vi "GraphForm (SubVI) 16.vi"() -> ()   [LabVIEW 2013]
uses:
  Global R.vi
  Global T.vi
panel:
  in  "9_ch_visible":bool=TRUE
  out "T15":dbl format="%.2f"
  out "T13":dbl format="%.2f"
  out "T16":dbl format="%.2f"
  out "T14":dbl format="%.2f"
  out "T11":dbl format="%.2f"
  out "T9":dbl format="%.2f"
  out "T12":dbl format="%.2f"
  out "T10":dbl format="%.2f"
  in  "10_ch_visible":bool=TRUE
  in  "11_ch_visible":bool=TRUE
  in  "12_ch_visible":bool=TRUE
  in  "13_ch_visible":bool=TRUE
  in  "14_ch_visible":bool=TRUE
  in  "15_ch_visible":bool=TRUE
  in  "16_ch_visible":bool=TRUE
  in  "1_ch_visible":bool=TRUE
  out "T7":dbl format="%.2f"
  out "T5":dbl format="%.2f"
  out "T8":dbl format="%.2f"
  out "T6":dbl format="%.2f"
  out "T3":dbl format="%.2f"
  out "T1":dbl format="%.2f"
  out "T4":dbl format="%.2f"
  out "T2":dbl format="%.2f"
  in  "R":T1
  in  "stop":bool
  in  "T":T2
  in  "Title":string
  out "часы":string="0"
  in  "Добавить время":dbl(ring)=300.0 items=["1 мин."=60.0, "5 мин."=300.0, "20 мин."=1200.0]
  out "мин.":string="1"
  in  "xScale +":bool
  in  "xScale -":bool
  in  "Autoscale":bool=TRUE
  in  "R max":u16=6000 min=2 max=10000 step=1
  in  "R min":u16=100 min=1 max=350
  in  "Т max":u16=300 min=2 max=500 step=1
  in  "Т min":u16=3 min=1 max=350
  in  "2_ch_visible":bool=TRUE
  in  "3_ch_visible":bool=TRUE
  in  "4_ch_visible":bool=TRUE
  in  "5_ch_visible":bool=TRUE
  in  "6_ch_visible":bool=TRUE
  in  "7_ch_visible":bool=TRUE
  in  "8_ch_visible":bool=TRUE
  out "Graphs T":dynamicdata(graph)
  out "Graphs R":dynamicdata(graph)
  # "№"
  # "№"
  # "T [К]"
  # "T [К]"
  # "1"
  # "9"
  # "2"
  # "10"
  # "3"
  # "11"
  # "4"
  # "12"
  # "5"
  # "13"
  # "6"
  # "14"
  # "7"
  # "15"
  # "8"
  # "16"
  # "Интервал просмотра"
  # ":"
  # "Шкала R"
  # "Шкала Т"
  # "Температура, К"
  # "Сопротивление, Ом"
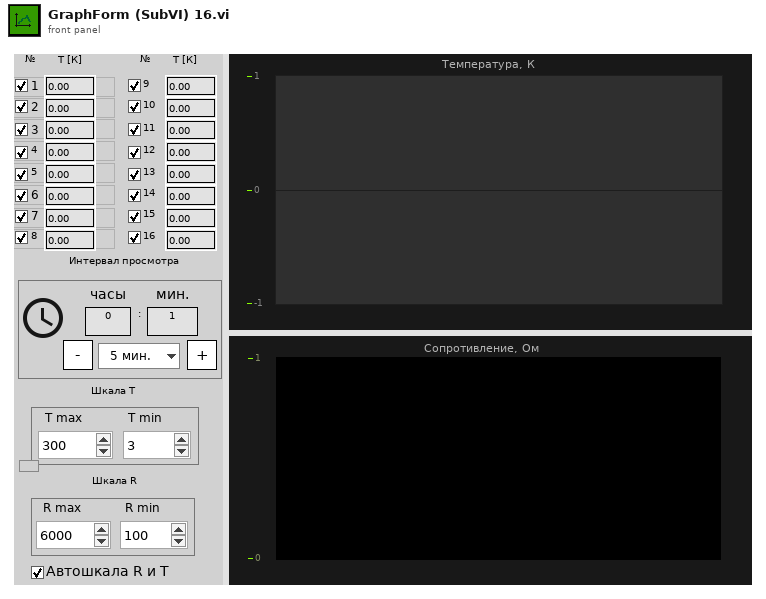
[diagram p1: front panel]
types:
  T1 = cluster{" R1":dbl, " R2":dbl, " R3":dbl, " R4":dbl, " R5":dbl, "R6":dbl, " R7":dbl, "R8":dbl, "R16":dbl, " R15":dbl, "R14":dbl, " R13":dbl, " R12":dbl, " R11":dbl, " R10":dbl, " R9":dbl}
  T2 = cluster{" T1":dbl, " T2":dbl, " T3":dbl, " T4":dbl, " T5":dbl, "T6":dbl, " T7":dbl, "T8":dbl, "T16":dbl, " T15":dbl, "T14":dbl, " T13":dbl, " T12":dbl, " T11":dbl, " T10":dbl, " T9":dbl}
  T3 = cluster{"1":dbl, " 2":dbl, " 3":dbl, "4":dbl, "5":dbl, "6":dbl, "7":dbl, "8":dbl, "9":dbl, " 10":dbl, " 11":dbl, "12":dbl, "13":dbl, "14":dbl, "15":dbl, "16":dbl}
  T4 = cluster{bool, bool, bool, bool, bool, bool, bool, bool, bool, bool, bool, bool, bool, bool, bool, bool}
  T5 = typedef "LVDateTimeRec.ctl" = cluster{"fractional second":dbl, "second":i32, "minute":i32, "hour":i32, "day of month":i32, "month":i32, "year":i32, "day of week":i32, "day of year":i32, "DST":i32}
  T6 = cluster{"1":dbl, " 2":dbl, " 3":dbl, "4":dbl, "5":dbl, "6":dbl, "7":dbl, "8":dbl, "1 2":dbl, " 10":dbl, " 11":dbl, "12":dbl, "13":dbl, "14":dbl, "15":dbl, "16":dbl}
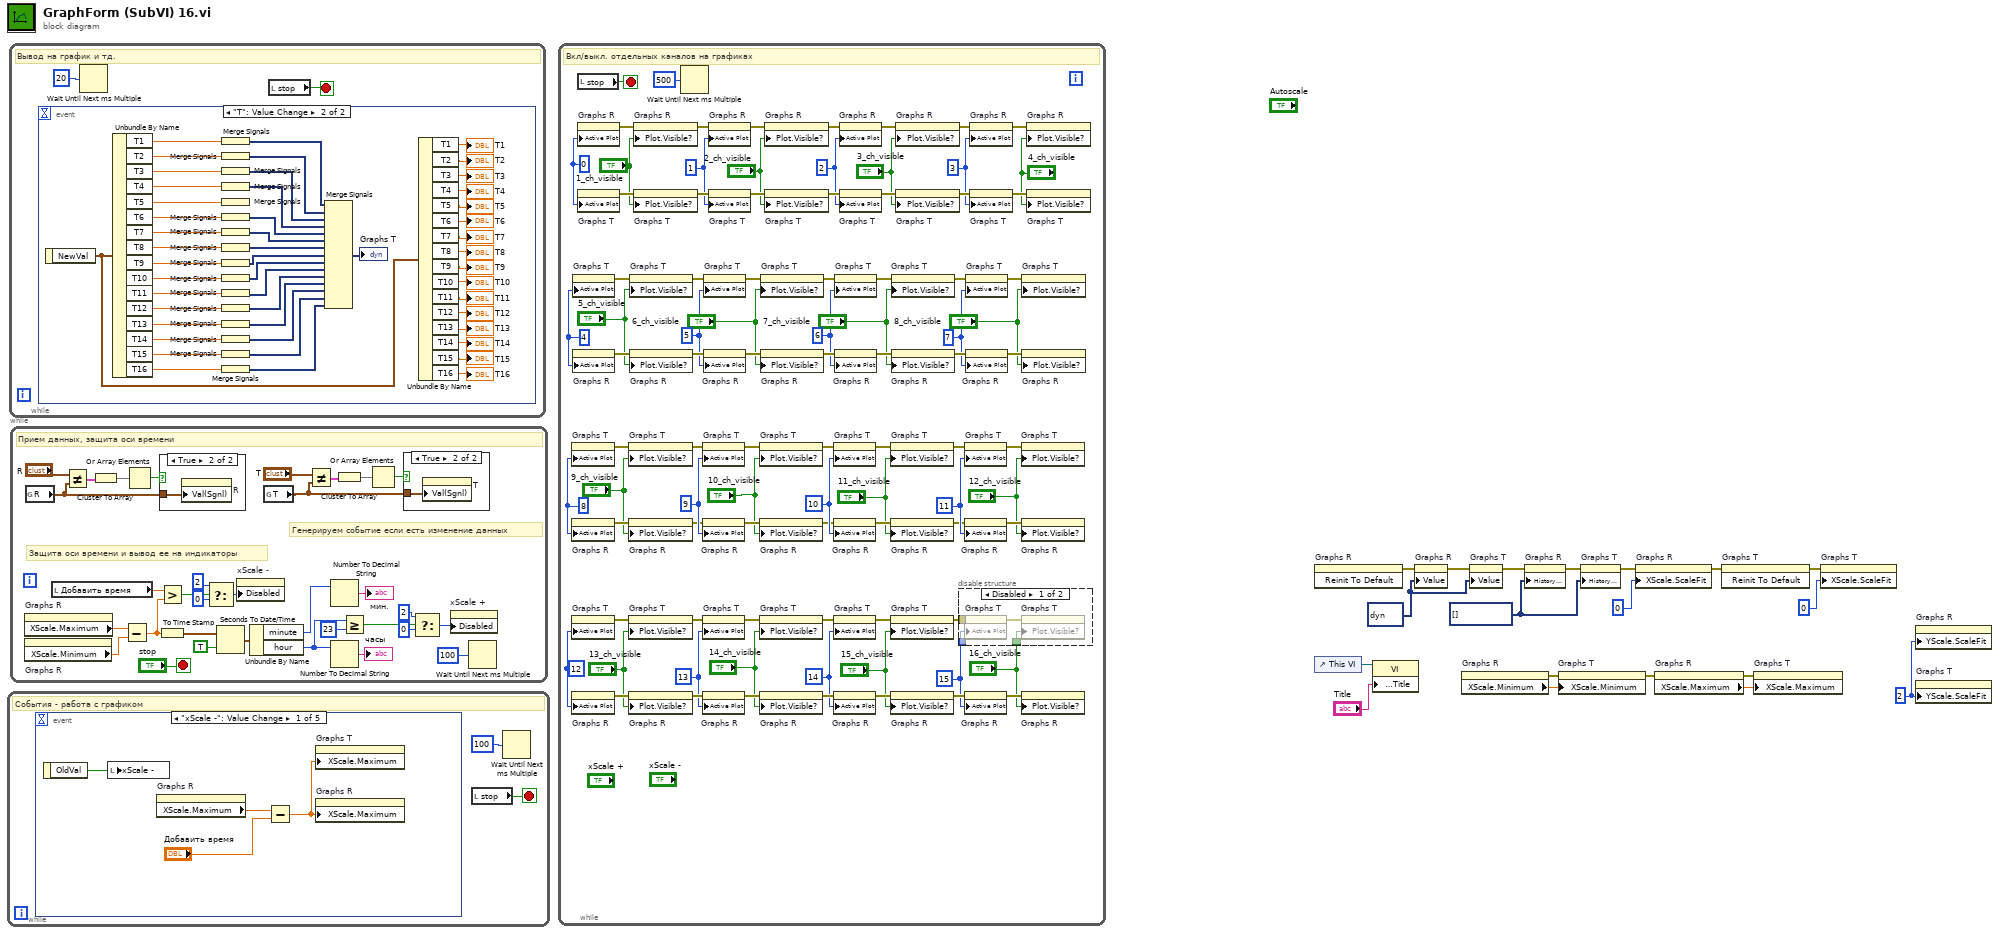
[diagram p0: block diagram]
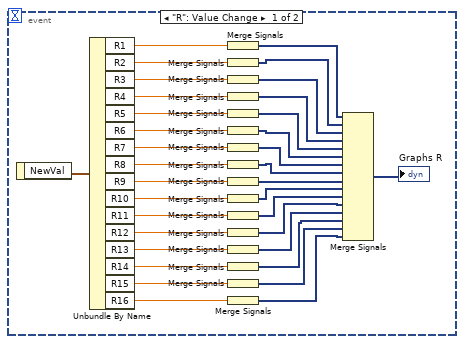
[diagram p3: hidden frame]
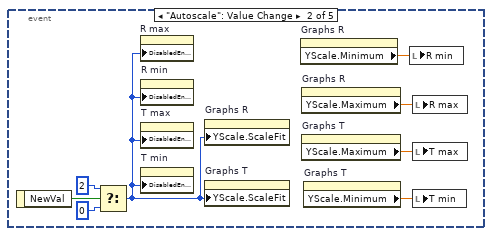
[diagram p6: hidden frame]
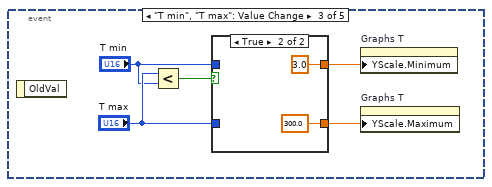
[diagram p7: hidden frame]
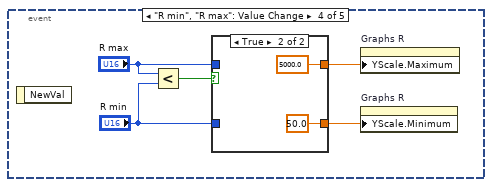
[diagram p9: hidden frame]
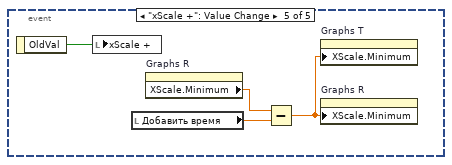
[diagram p11: hidden frame]
diagram:
  w3 = u8 2 ("Y Scale.Scale Fit")
  w14 = dynamicdata[] [] ("History Data")
  w15 = dynamicdata [{"t0"=timestamp(3465273261.7246556 s since 1904-01-01), "dt"=1.0, "Y"=[0.1931097262457384]}, {"t0"=timestamp(3465273261.7246556 s since 1904-01-01), "dt"=1.0, "Y"=[0.3594116459482981]}, {"t0"=timestamp(3465273261.7246556 s since 1904-01-01), "dt"=1.0, "Y"=[0.8898205452798131]}, {"t0"=timestamp(3465273261.7246556 s since 1904-01-01), "dt"=1.0, "Y"=[0.747699236883661]}] ("Graphs")
  n1 = while {
    stop <- w20 stop-if-true
    # "События - работа с графиком"
    n2 = event shown="[0] \"xScale -\": Value Change" {
      selector: _ -> [_ _ _ _ _]
      dyn-events: _ -> [_ _ _ _ _]
      timeout: _ -> [_ _ _ _ _]
      event "xScale -": Value Change {
        n3 = event-data() -> ("OldVal"=w25:bool)  [unwired: 1 in]
        n4 = local write "xScale -"(w25) -> ()
        n5 = property on="Graphs R" class="WFChart (strict)"() -> ("XScale.Maximum"=w23:dbl)  [unwired: 2 in, 2 out]
        n6 = Subtract(x=w23, y="Добавить время") -> (x-y=w24:dbl)
        n7 = property on="Graphs T" class="WFChart (strict)"("XScale.Maximum"=w24) -> ()  [unwired: 2 in, 2 out]
        n8 = property on="Graphs R" class="WFChart (strict)"("XScale.Maximum"=w24) -> ()  [unwired: 2 in, 2 out]
      }
      event "Autoscale": Value Change {
        n9 = event-data() -> ("NewVal"=w26:bool)  [unwired: 1 in]
        n10 = Select(t=u8 2 ("Y Scale.Scale Fit"), s=w26, f=u8 0 ("Y Scale.Scale Fit")) -> (s? t:f=w29:u8)
        n11 = property on="R max" class="DigNum (strict)"("DisabledEnum"=w29) -> ()  [unwired: 2 in, 2 out]
        n12 = property on="R min" class="DigNum (strict)"("DisabledEnum"=w29) -> ()  [unwired: 2 in, 2 out]
        n13 = property on="Т max" class="DigNum (strict)"("DisabledEnum"=w29) -> ()  [unwired: 2 in, 2 out]
        n14 = property on="Т min" class="DigNum (strict)"("DisabledEnum"=w29) -> ()  [unwired: 2 in, 2 out]
        n15 = property on="Graphs R" class="WFChart (strict)"("YScale.ScaleFit"=w29) -> ()  [unwired: 2 in, 2 out]
        n16 = property on="Graphs T" class="WFChart (strict)"("YScale.ScaleFit"=w29) -> ()  [unwired: 2 in, 2 out]
        n17 = property on="Graphs R" class="WFChart (strict)"() -> ("YScale.Minimum"=w30:dbl)  [unwired: 2 in, 2 out]
        n18 = property on="Graphs R" class="WFChart (strict)"() -> ("YScale.Maximum"=w31:dbl)  [unwired: 2 in, 2 out]
        n19 = property on="Graphs T" class="WFChart (strict)"() -> ("YScale.Maximum"=w33:dbl)  [unwired: 2 in, 2 out]
        n20 = property on="Graphs T" class="WFChart (strict)"() -> ("YScale.Minimum"=w32:dbl)  [unwired: 2 in, 2 out]
        n21 = local write "R min"(w30) -> ()
        n22 = local write "R max"(w31) -> ()
        n23 = local write "Т max"(w33) -> ()
        n24 = local write "Т min"(w32) -> ()
      }
      event "Т min", "Т max": Value Change {
        n25 = event-data() -> ()  [unwired: 1 in, 1 out]
        n26 = Less?(x="Т max", y="Т min") -> (x < y?=w36:bool)
        n27 = case shown="True" w36 {
          tunnel: [w39 300.0 ("x+1")] -> w38
          tunnel: [w40 3.0 ("x+1")] -> w37
          tunnel: "Т max" -> [w39 _]
          tunnel: "Т min" -> [w40 _]
          frame False {
          }
          frame True {
          }
        }
        n28 = property on="Graphs T" class="WFChart (strict)"("YScale.Minimum"=w37) -> ()  [unwired: 2 in, 2 out]
        n29 = property on="Graphs T" class="WFChart (strict)"("YScale.Maximum"=w38) -> ()  [unwired: 2 in, 2 out]
      }
      event "R min", "R max": Value Change {
        n30 = event-data() -> ()  [unwired: 1 in, 1 out]
        n31 = Less?(x="R max", y="R min") -> (x < y?=w47:bool)
        n32 = case shown="True" w47 {
          tunnel: [w48 5000.0 ("x+1")] -> w43
          tunnel: [w49 50.0 ("x+1")] -> w44
          tunnel: "R max" -> [w48 _]
          tunnel: "R min" -> [w49 _]
          frame False {
          }
          frame True {
          }
        }
        n33 = property on="Graphs R" class="WFChart (strict)"("YScale.Maximum"=w43) -> ()  [unwired: 2 in, 2 out]
        n34 = property on="Graphs R" class="WFChart (strict)"("YScale.Minimum"=w44) -> ()  [unwired: 2 in, 2 out]
      }
      event "xScale +": Value Change {
        n35 = event-data() -> ("OldVal"=w55:bool)  [unwired: 1 in]
        n36 = local write "xScale +"(w55) -> ()
        n37 = local read "Добавить время"() -> (w52:dbl)
        n38 = property on="Graphs R" class="WFChart (strict)"() -> ("XScale.Minimum"=w53:dbl)  [unwired: 2 in, 2 out]
        n39 = Subtract(x=w53, y=w52) -> (x-y=w54:dbl)
        n40 = property on="Graphs T" class="WFChart (strict)"("XScale.Minimum"=w54) -> ()  [unwired: 2 in, 2 out]
        n41 = property on="Graphs R" class="WFChart (strict)"("XScale.Minimum"=w54) -> ()  [unwired: 2 in, 2 out]
      }
    }
    n42 = local read "stop"() -> (w20:bool)
    n43 = Wait Until Next ms Multiple(millisecond multiple=u32 100) -> ()  [unwired: 1 out]
  }
  n44 = while {
    stop <- w56 stop-if-true
    # "Вывод на график и тд."
    n45 = event shown="[1] \"T\": Value Change" {
      selector: _ -> [_ _]
      dyn-events: _ -> [_ _]
      timeout: _ -> [_ _]
      event "R": Value Change {
        n46 = event-data() -> ("NewVal"=w91:T1)  [unwired: 1 in]
        n47 = Unbundle By Name(w91) -> ("R1"=w90:dbl, "R2"=w89:dbl, "R3"=w88:dbl, "R4"=w87:dbl, "R5"=w86:dbl, "R6"=w85:dbl, "R7"=w84:dbl, "R8"=w83:dbl, "R9"=w82:dbl, "R10"=w81:dbl, "R11"=w80:dbl, "R12"=w79:dbl, "R13"=w78:dbl, "R14"=w77:dbl, "R15"=w76:dbl, "R16"=w75:dbl)
        n48 = Merge Signals(w90) -> (w74:dynamicdata)
        n49 = Merge Signals(w89) -> (w73:dynamicdata)
        n50 = Merge Signals(w88) -> (w72:dynamicdata)
        n51 = Merge Signals(w87) -> (w71:dynamicdata)
        n52 = Merge Signals(w86) -> (w70:dynamicdata)
        n53 = Merge Signals(w85) -> (w69:dynamicdata)
        n54 = Merge Signals(w84) -> (w68:dynamicdata)
        n55 = Merge Signals(w83) -> (w67:dynamicdata)
        n56 = Merge Signals(w82) -> (w66:dynamicdata)
        n57 = Merge Signals(w81) -> (w65:dynamicdata)
        n58 = Merge Signals(w80) -> (w64:dynamicdata)
        n59 = Merge Signals(w79) -> (w63:dynamicdata)
        n60 = Merge Signals(w78) -> (w62:dynamicdata)
        n61 = Merge Signals(w77) -> (w61:dynamicdata)
        n62 = Merge Signals(w76) -> (w60:dynamicdata)
        n63 = Merge Signals(w75) -> (w59:dynamicdata)
        n64 = Merge Signals(w74, w73, w72, w71, w70, w69, w68, w67, w66, w65, w64, w63, w62, w61, w60, w59) -> (→"Graphs R":dynamicdata)
      }
      event "T": Value Change {
        n65 = event-data() -> ("NewVal"=w108:T2)  [unwired: 1 in]
        n66 = Unbundle By Name(w108) -> ("T1"=w140:dbl, "T2"=w139:dbl, "T3"=w138:dbl, "T4"=w137:dbl, "T5"=w136:dbl, "T6"=w135:dbl, "T7"=w134:dbl, "T8"=w133:dbl, "T9"=w132:dbl, "T10"=w131:dbl, "T11"=w130:dbl, "T12"=w129:dbl, "T13"=w128:dbl, "T14"=w127:dbl, "T15"=w126:dbl, "T16"=w125:dbl)
        n67 = Merge Signals(w140) -> (w124:dynamicdata)
        n68 = Merge Signals(w139) -> (w123:dynamicdata)
        n69 = Merge Signals(w138) -> (w112:dynamicdata)
        n70 = Merge Signals(w137) -> (w122:dynamicdata)
        n71 = Merge Signals(w136) -> ()  [unwired: 1 out]
        n72 = Merge Signals(w135) -> (w121:dynamicdata)
        n73 = Merge Signals(w134) -> (w120:dynamicdata)
        n74 = Merge Signals(w133) -> (w119:dynamicdata)
        n75 = Merge Signals(w132) -> (w118:dynamicdata)
        n76 = Merge Signals(w131) -> (w117:dynamicdata)
        n77 = Merge Signals(w130) -> (w111:dynamicdata)
        n78 = Merge Signals(w129) -> (w110:dynamicdata)
        n79 = Merge Signals(w128) -> (w116:dynamicdata)
        n80 = Merge Signals(w127) -> (w115:dynamicdata)
        n81 = Merge Signals(w126) -> (w114:dynamicdata)
        n82 = Merge Signals(w125) -> (w113:dynamicdata)
        n83 = Merge Signals(w124, w123, w112, w122, w121, w120, w119, w118, w117, w111, w110, w116, w115, w114, w113) -> (→"Graphs T":dynamicdata)
        n84 = Unbundle By Name(w108) -> ("T1"=→"T1":dbl, "T2"=→"T2":dbl, "T3"=→"T3":dbl, "T4"=→"T4":dbl, "T5"=→"T5":dbl, "T6"=→"T6":dbl, "T7"=→"T7":dbl, "T8"=→"T8":dbl, "T9"=→"T9":dbl, "T10"=→"T10":dbl, "T11"=→"T11":dbl, "T12"=→"T12":dbl, "T13"=→"T13":dbl, "T14"=→"T14":dbl, "T15"=→"T15":dbl, "T16"=→"T16":dbl)
      }
    }
    n85 = Wait Until Next ms Multiple(millisecond multiple=u32 20) -> ()  [unwired: 1 out]
    n86 = local read "stop"() -> (w56:bool)
  }
  n87 = while {
    stop <- "stop" stop-if-true
    # "Генерируем событие если есть изменение данных"
    # "Защита оси времени и вывод ее на индикаторы"
    # "Прием данных, защита оси времени"
    n88 = property on="Graphs R" class="WFChart (strict)"() -> ("XScale.Maximum"=w172:dbl)  [unwired: 2 in, 2 out]
    n89 = property on="Graphs R" class="WFChart (strict)"() -> ("XScale.Minimum"=w171:dbl)  [unwired: 2 in, 2 out]
    n90 = global read "Global R.vi" "R"() -> (w158:T3)
    n91 = local read "Добавить время"() -> (w170:dbl)
    n92 = Not Equal?(x="R", y=w158) -> (x != y?=w155:T4)
    n93 = Cluster To Array(cluster=w155) -> (array=w156:bool[])
    n94 = Subtract(x=w172, y=w171) -> (x-y=w165:dbl)
    n95 = Or Array Elements(Boolean array=w156) -> (logical OR=w157:bool)
    n96 = Greater?(x=w170, y=w165) -> (0:w154:bool)
    n97 = To Time Stamp(1:w165) -> (0:w168:timestamp)
    n98 = case shown="True" w157 {
      tunnel: w158 -> [_ w174]
      frame False {
      }
      frame True {
        n99 = property on="R" class="Clust (strict)"("Val(Sgnl)"=w174) -> ()  [unwired: 2 in, 2 out]
      }
    }
    n100 = Select(t=u8 2 ("Disabled"), s=w154, f=u8 0 ("Disabled")) -> (s? t:f=w153:u8)
    n101 = Seconds To Date/Time(time stamp (now)=w168, to UTC (F)=TRUE) -> (date time rec=w167:T5)
    n102 = property on="xScale -" class="Bool (strict)"("Disabled"=w153) -> ()  [unwired: 2 in, 2 out]
    n103 = Unbundle By Name(w167) -> ("minute"=w166:i32, "hour"=w164:i32)
    n104 = global read "Global T.vi" "T"() -> (w141:T6)
    n105 = Not Equal?(x="T", y=w141) -> (x != y?=w146:T4)
    n106 = Number To Decimal String(number=w166) -> (decimal integer string=→"мин.":string)  [unwired: 1 out]
    n107 = Number To Decimal String(number=w164) -> (decimal integer string=→"часы":string)  [unwired: 1 out]
    n108 = Cluster To Array(cluster=w146) -> (array=w145:bool[])
    n109 = Greater Or Equal?(x=w164, y=23) -> (x >= y?=w149:bool)
    n110 = Or Array Elements(Boolean array=w145) -> (logical OR=w144:bool)
    n111 = case shown="True" w144 {
      tunnel: w141 -> [_ w173]
      frame False {
      }
      frame True {
        n112 = property on="T" class="Clust (strict)"("Val(Sgnl)"=w173) -> ()  [unwired: 2 in, 2 out]
      }
    }
    n113 = Select(t=u8 2 ("Disabled"), s=w149, f=u8 0 ("Disabled")) -> (s? t:f=w147:u8)
    n114 = property on="xScale +" class="Bool (strict)"("Disabled"=w147) -> ()  [unwired: 2 in, 2 out]
    n115 = Wait Until Next ms Multiple(millisecond multiple=u32 100) -> ()  [unwired: 1 out]
  }
  n116 = while {
    stop <- w218 stop-if-true
    w180 = u32 15 ("Active Plot")
    w181 = u32 14 ("Active Plot")
    w182 = u32 13 ("Active Plot")
    w179 = u32 12 ("Active Plot")
    w217 = u32 11 ("Active Plot")
    w216 = u32 10 ("Active Plot")
    w215 = u32 9 ("Active Plot")
    w214 = u32 8 ("Active Plot")
    w220 = u32 7 ("Active Plot")
    w222 = u32 6 ("Active Plot")
    w224 = u32 5 ("Active Plot")
    w226 = u32 4 ("Active Plot")
    w236 = u32 3 ("Active Plot")
    w239 = u32 2 ("Active Plot")
    w242 = u32 1 ("Active Plot")
    w247 = u32 0 ("Active Plot")
    # "Вкл/выкл. отдельных каналов на графиках"
    n117 = property on="Graphs T" class="WFChart (strict)"("Active Plot"=w214) -> (error out=w200:errorcluster)  [unwired: 2 in, 1 out]
    n118 = property on="Graphs R" class="WFChart (strict)"("Active Plot"=w214) -> (error out=w213:errorcluster)  [unwired: 2 in, 1 out]
    n119 = property on="Graphs T" class="WFChart (strict)"("Active Plot"=w179) -> (error out=w195:errorcluster)  [unwired: 2 in, 1 out]
    n120 = property on="Graphs R" class="WFChart (strict)"("Active Plot"=w179) -> (error out=w183:errorcluster)  [unwired: 2 in, 1 out]
    n121 = property on="Graphs T" class="WFChart (strict)"("Active Plot"=w226) -> (error out=w258:errorcluster)  [unwired: 2 in, 1 out]
    n122 = property on="Graphs R" class="WFChart (strict)"("Active Plot"=w226) -> (error out=w227:errorcluster)  [unwired: 2 in, 1 out]
    n123 = local read "stop"() -> (w218:bool)
    n124 = property on="Graphs R" class="WFChart (strict)"("Active Plot"=w247) -> (error out=w248:errorcluster)  [unwired: 2 in, 1 out]
    n125 = property on="Graphs T" class="WFChart (strict)"("Active Plot"=w247) -> (error out=w259:errorcluster)  [unwired: 2 in, 1 out]
    n126 = property on="Graphs T" class="WFChart (strict)"(error in=w200, "Plot.Visible?"="9_ch_visible") -> (error out=w202:errorcluster)  [unwired: 1 in, 1 out]
    n127 = property on="Graphs R" class="WFChart (strict)"(error in=w213, "Plot.Visible?"="9_ch_visible") -> (error out=w209:errorcluster)  [unwired: 1 in, 1 out]
    n128 = property on="Graphs T" class="WFChart (strict)"(error in=w195, "Plot.Visible?"="13_ch_visible") -> (error out=w193:errorcluster)  [unwired: 1 in, 1 out]
    n129 = property on="Graphs R" class="WFChart (strict)"(error in=w183, "Plot.Visible?"="13_ch_visible") -> (error out=w187:errorcluster)  [unwired: 1 in, 1 out]
    n130 = property on="Graphs T" class="WFChart (strict)"(error in=w258, "Plot.Visible?"="5_ch_visible") -> (error out=w256:errorcluster)  [unwired: 1 in, 1 out]
    n131 = property on="Graphs R" class="WFChart (strict)"(error in=w227, "Plot.Visible?"="5_ch_visible") -> (error out=w231:errorcluster)  [unwired: 1 in, 1 out]
    n132 = property on="Graphs R" class="WFChart (strict)"(error in=w248, "Plot.Visible?"="1_ch_visible") -> (error out=w241:errorcluster)  [unwired: 1 in, 1 out]
    n133 = property on="Graphs T" class="WFChart (strict)"(error in=w259, "Plot.Visible?"="1_ch_visible") -> (error out=w261:errorcluster)  [unwired: 1 in, 1 out]
    n134 = Wait Until Next ms Multiple(millisecond multiple=u32 500) -> ()  [unwired: 1 out]
    n135 = property on="Graphs T" class="WFChart (strict)"(error in=w202, "Active Plot"=w215) -> (error out=w201:errorcluster)  [unwired: 1 in, 1 out]
    n136 = property on="Graphs R" class="WFChart (strict)"(error in=w209, "Active Plot"=w215) -> (error out=w212:errorcluster)  [unwired: 1 in, 1 out]
    n137 = property on="Graphs T" class="WFChart (strict)"(error in=w193, "Active Plot"=w182) -> (error out=w194:errorcluster)  [unwired: 1 in, 1 out]
    n138 = property on="Graphs R" class="WFChart (strict)"(error in=w187, "Active Plot"=w182) -> (error out=w184:errorcluster)  [unwired: 1 in, 1 out]
    n139 = property on="Graphs T" class="WFChart (strict)"(error in=w256, "Active Plot"=w224) -> (error out=w257:errorcluster)  [unwired: 1 in, 1 out]
    n140 = property on="Graphs R" class="WFChart (strict)"(error in=w231, "Active Plot"=w224) -> (error out=w228:errorcluster)  [unwired: 1 in, 1 out]
    n141 = property on="Graphs R" class="WFChart (strict)"(error in=w241, "Active Plot"=w242) -> (error out=w245:errorcluster)  [unwired: 1 in, 1 out]
    n142 = property on="Graphs T" class="WFChart (strict)"(error in=w261, "Active Plot"=w242) -> (error out=w260:errorcluster)  [unwired: 1 in, 1 out]
    n143 = property on="Graphs T" class="WFChart (strict)"(error in=w201, "Plot.Visible?"="10_ch_visible") -> (error out=w204:errorcluster)  [unwired: 1 in, 1 out]
    n144 = property on="Graphs R" class="WFChart (strict)"(error in=w212, "Plot.Visible?"="10_ch_visible") -> (error out=w208:errorcluster)  [unwired: 1 in, 1 out]
    n145 = property on="Graphs T" class="WFChart (strict)"(error in=w194, "Plot.Visible?"="14_ch_visible") -> (error out=w191:errorcluster)  [unwired: 1 in, 1 out]
    n146 = property on="Graphs R" class="WFChart (strict)"(error in=w184, "Plot.Visible?"="14_ch_visible") -> (error out=w188:errorcluster)  [unwired: 1 in, 1 out]
    n147 = property on="Graphs T" class="WFChart (strict)"(error in=w257, "Plot.Visible?"="6_ch_visible") -> (error out=w254:errorcluster)  [unwired: 1 in, 1 out]
    n148 = property on="Graphs R" class="WFChart (strict)"(error in=w228, "Plot.Visible?"="6_ch_visible") -> (error out=w232:errorcluster)  [unwired: 1 in, 1 out]
    n149 = property on="Graphs R" class="WFChart (strict)"(error in=w245, "Plot.Visible?"="2_ch_visible") -> (error out=w238:errorcluster)  [unwired: 1 in, 1 out]
    n150 = property on="Graphs T" class="WFChart (strict)"(error in=w260, "Plot.Visible?"="2_ch_visible") -> (error out=w262:errorcluster)  [unwired: 1 in, 1 out]
    n151 = property on="Graphs T" class="WFChart (strict)"(error in=w204, "Active Plot"=w216) -> (error out=w203:errorcluster)  [unwired: 1 in, 1 out]
    n152 = property on="Graphs R" class="WFChart (strict)"(error in=w208, "Active Plot"=w216) -> (error out=w211:errorcluster)  [unwired: 1 in, 1 out]
    n153 = property on="Graphs T" class="WFChart (strict)"(error in=w191, "Active Plot"=w181) -> (error out=w192:errorcluster)  [unwired: 1 in, 1 out]
    n154 = property on="Graphs R" class="WFChart (strict)"(error in=w188, "Active Plot"=w181) -> (error out=w185:errorcluster)  [unwired: 1 in, 1 out]
    n155 = property on="Graphs T" class="WFChart (strict)"(error in=w254, "Active Plot"=w222) -> (error out=w255:errorcluster)  [unwired: 1 in, 1 out]
    n156 = property on="Graphs R" class="WFChart (strict)"(error in=w232, "Active Plot"=w222) -> (error out=w229:errorcluster)  [unwired: 1 in, 1 out]
    n157 = property on="Graphs R" class="WFChart (strict)"(error in=w238, "Active Plot"=w239) -> (error out=w244:errorcluster)  [unwired: 1 in, 1 out]
    n158 = property on="Graphs T" class="WFChart (strict)"(error in=w262, "Active Plot"=w239) -> (error out=w249:errorcluster)  [unwired: 1 in, 1 out]
    n159 = property on="Graphs T" class="WFChart (strict)"(error in=w203, "Plot.Visible?"="11_ch_visible") -> (error out=w206:errorcluster)  [unwired: 1 in, 1 out]
    n160 = property on="Graphs R" class="WFChart (strict)"(error in=w211, "Plot.Visible?"="11_ch_visible") -> (error out=w207:errorcluster)  [unwired: 1 in, 1 out]
    n161 = property on="Graphs T" class="WFChart (strict)"(error in=w192, "Plot.Visible?"="15_ch_visible") -> (error out=w190:errorcluster)  [unwired: 1 in, 1 out]
    n162 = property on="Graphs R" class="WFChart (strict)"(error in=w185, "Plot.Visible?"="15_ch_visible") -> (error out=w189:errorcluster)  [unwired: 1 in, 1 out]
    n163 = property on="Graphs T" class="WFChart (strict)"(error in=w255, "Plot.Visible?"="7_ch_visible") -> (error out=w252:errorcluster)  [unwired: 1 in, 1 out]
    n164 = property on="Graphs R" class="WFChart (strict)"(error in=w229, "Plot.Visible?"="7_ch_visible") -> (error out=w233:errorcluster)  [unwired: 1 in, 1 out]
    n165 = property on="Graphs R" class="WFChart (strict)"(error in=w244, "Plot.Visible?"="3_ch_visible") -> (error out=w235:errorcluster)  [unwired: 1 in, 1 out]
    n166 = property on="Graphs T" class="WFChart (strict)"(error in=w249, "Plot.Visible?"="3_ch_visible") -> (error out=w250:errorcluster)  [unwired: 1 in, 1 out]
    n167 = disable-structure shown="Disabled" {
      disable-tunnel: w190 -> [w266 _]
      disable-tunnel: w180 -> [w265 _]
      disable-tunnel: "16_ch_visible" -> [w264 _]
      frame Disabled {
        n168 = property on="Graphs T" class="WFChart (strict)"(error in=w266, "Active Plot"=w265) -> (error out=w267:errorcluster)  [unwired: 1 in, 1 out]
        n169 = property on="Graphs T" class="WFChart (strict)"(error in=w267, "Plot.Visible?"=w264) -> ()  [unwired: 1 in, 2 out]
      }
      frame Enabled {
      }
    }
    n170 = property on="Graphs T" class="WFChart (strict)"(error in=w206, "Active Plot"=w217) -> (error out=w205:errorcluster)  [unwired: 1 in, 1 out]
    n171 = property on="Graphs R" class="WFChart (strict)"(error in=w207, "Active Plot"=w217) -> (error out=w210:errorcluster)  [unwired: 1 in, 1 out]
    n172 = property on="Graphs R" class="WFChart (strict)"(error in=w189, "Active Plot"=w180) -> (error out=w186:errorcluster)  [unwired: 1 in, 1 out]
    n173 = property on="Graphs T" class="WFChart (strict)"(error in=w252, "Active Plot"=w220) -> (error out=w253:errorcluster)  [unwired: 1 in, 1 out]
    n174 = property on="Graphs R" class="WFChart (strict)"(error in=w233, "Active Plot"=w220) -> (error out=w230:errorcluster)  [unwired: 1 in, 1 out]
    n175 = property on="Graphs R" class="WFChart (strict)"(error in=w235, "Active Plot"=w236) -> (error out=w243:errorcluster)  [unwired: 1 in, 1 out]
    n176 = property on="Graphs T" class="WFChart (strict)"(error in=w250, "Active Plot"=w236) -> (error out=w251:errorcluster)  [unwired: 1 in, 1 out]
    n177 = property on="Graphs T" class="WFChart (strict)"(error in=w205, "Plot.Visible?"="12_ch_visible") -> ()  [unwired: 1 in, 2 out]
    n178 = property on="Graphs R" class="WFChart (strict)"(error in=w210, "Plot.Visible?"="12_ch_visible") -> ()  [unwired: 1 in, 2 out]
    n179 = property on="Graphs R" class="WFChart (strict)"(error in=w186, "Plot.Visible?"="16_ch_visible") -> ()  [unwired: 1 in, 2 out]
    n180 = property on="Graphs T" class="WFChart (strict)"(error in=w253, "Plot.Visible?"="8_ch_visible") -> ()  [unwired: 1 in, 2 out]
    n181 = property on="Graphs R" class="WFChart (strict)"(error in=w230, "Plot.Visible?"="8_ch_visible") -> ()  [unwired: 1 in, 2 out]
    n182 = property on="Graphs R" class="WFChart (strict)"(error in=w243, "Plot.Visible?"="4_ch_visible") -> ()  [unwired: 1 in, 2 out]
    n183 = property on="Graphs T" class="WFChart (strict)"(error in=w251, "Plot.Visible?"="4_ch_visible") -> ()  [unwired: 1 in, 2 out]
  }
  n184 = invoke on="Graphs R" class="WFChart (strict)" method="Reinit To Default"() -> (error out=w19:errorcluster)  [unwired: 3 in, 2 out]
  n185 = control-ref of="This VI"() -> (w2:refnum<vi>)
  n186 = property class="VI"(reference=w2, "Front Panel.Title"="Title") -> ()  [unwired: 1 in, 2 out]
  n187 = property on="Graphs R" class="WFChart (strict)"(error in=w19, "Value"=w15) -> (error out=w13:errorcluster)  [unwired: 1 in, 1 out]
  n188 = property on="Graphs R" class="WFChart (strict)"() -> (error out=w5:errorcluster, "XScale.Minimum"=w8:dbl)  [unwired: 2 in, 1 out]
  n189 = property on="Graphs T" class="WFChart (strict)"(error in=w13, "Value"=w15) -> (error out=w12:errorcluster)  [unwired: 1 in, 1 out]
  n190 = property on="Graphs R" class="WFChart (strict)"(error in=w12, "History Data"=w14) -> (error out=w11:errorcluster)  [unwired: 1 in, 1 out]
  n191 = property on="Graphs T" class="WFChart (strict)"(error in=w5, "XScale.Minimum"=w8) -> (error out=w6:errorcluster)  [unwired: 1 in, 1 out]
  n192 = property on="Graphs T" class="WFChart (strict)"(error in=w11, "History Data"=w14) -> (error out=w10:errorcluster)  [unwired: 1 in, 1 out]
  n193 = property on="Graphs R" class="WFChart (strict)"(error in=w10, "XScale.ScaleFit"=u8 0 ("Y Scale.Scale Fit")) -> (error out=w17:errorcluster)  [unwired: 1 in, 1 out]
  n194 = property on="Graphs R" class="WFChart (strict)"(error in=w6) -> (error out=w4:errorcluster, "XScale.Maximum"=w7:dbl)  [unwired: 1 in, 1 out]
  n195 = invoke on="Graphs T" class="WFChart (strict)" method="Reinit To Default"(error in=w17) -> (error out=w9:errorcluster)  [unwired: 2 in, 2 out]
  n196 = property on="Graphs T" class="WFChart (strict)"(error in=w4, "XScale.Maximum"=w7) -> ()  [unwired: 1 in, 2 out]
  n197 = property on="Graphs T" class="WFChart (strict)"(error in=w9, "XScale.ScaleFit"=u8 0 ("Y Scale.Scale Fit")) -> ()  [unwired: 1 in, 2 out]
  n198 = property on="Graphs R" class="WFChart (strict)"("YScale.ScaleFit"=w3) -> ()  [unwired: 2 in, 2 out]
  n199 = property on="Graphs T" class="WFChart (strict)"("YScale.ScaleFit"=w3) -> ()  [unwired: 2 in, 2 out]
